vi "Register.vi"(8 "error in":errorcluster, 10 "TPCANHandle":T1 items=["PCAN_NONEBUS"=0, "PCAN_USBBUS1"=81, "PCAN_USBBUS2"=82, "PCAN_USBBUS3"=83, "PCAN_USBBUS4"=84, "PCAN_USBBUS5"=85, "PCAN_USBBUS6"=86, "PCAN_USBBUS7"=87, "PCAN_USBBUS8"=88, "PCAN_USBBUS9"=1289, "PCAN_USBBUS10"=1290, "PCAN_USBBUS11"=1291, "PCAN_USBBUS12"=1292, "PCAN_USBBUS13"=1293, "PCAN_USBBUS14"=1294, "PCAN_USBBUS15"=1295, "PCAN_USBBUS16"=1296], 11 "Win32 Event in":refnum<class "Win32 Event.lvclass">) -> (0 "error out":errorcluster, 3 "Win32 Event out":refnum<class "Win32 Event.lvclass">)   [LabVIEW 2019, in "PCANBasic.lvlib" / "Win32 Event.lvclass"]
uses:
  Win32 Event.lvclass
  TPCANHandle.ctl
  Win32 Event.lvclass/Win32 Event.ctl
  Set Receive Event.vi
  PCANBasic.lvlib
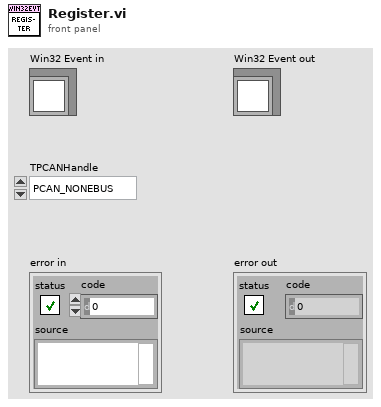
[diagram p1: front panel]
types:
  T1 = typedef "PCANBasic.lvlib/TPCANHandle.ctl" = u16
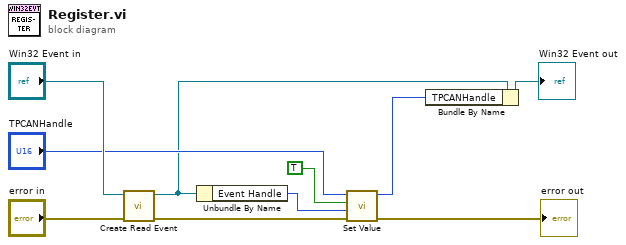
[diagram p0: block diagram]
diagram:
  n1 = call "Create Read Event.vi"("error in"="error in", "Win32 Event in"="Win32 Event in") -> ("error out"=w8:errorcluster, "Win32 Event out"=w3:refnum<class "Win32 Event.lvclass">)  [unwired: 8 in]
  n2 = Unbundle By Name(w3) -> ("Event Handle"=w2:u64)
  n3 = call-poly "Set Value.vi"("error in"=w8, "Event Handle"=w2, "Enable"=TRUE, "TPCANHandle in"="TPCANHandle") -> ("error out"=→"error out":errorcluster, "TPCANHandle out"=w4:T1)  [unwired: 5 in, 1 out]
  n4 = Bundle By Name(cluster=w3, "TPCANHandle"=w4) -> (→"Win32 Event out":refnum<class "Win32 Event.lvclass">)
